vi "Parameter to Value.vi"(8 "Memory":cluster{"w":i64, "x":i64, "y":i64, "z":i64}, 11 "Parameter":string) -> (3 "Value Out":i64)   [LabVIEW 2021]
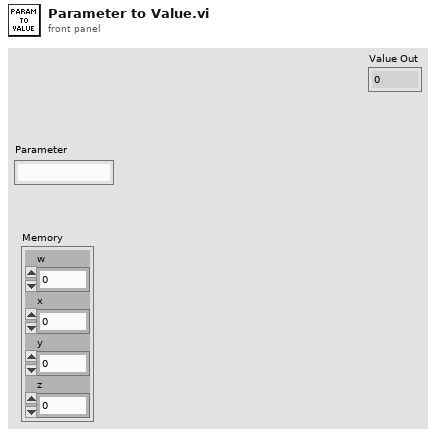
[diagram p1: front panel]
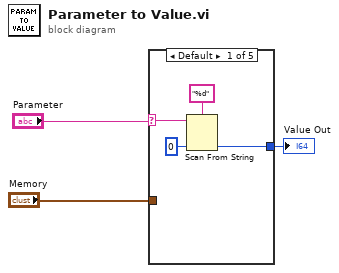
[diagram p0: block diagram]
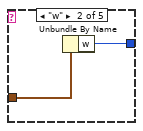
[diagram p2: hidden frame]
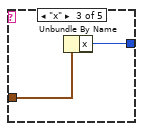
[diagram p3: hidden frame]
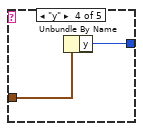
[diagram p4: hidden frame]
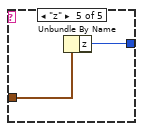
[diagram p5: hidden frame]
diagram:
  n1 = case shown="Default" "Parameter" {
    selector: "Parameter" -> [w7 _ _ _ _]
    tunnel: "Memory" -> [_ w9 w11 w13 w15]
    tunnel: [w4 w8 w10 w12 w14] -> w1
    frame Default {
      n2 = Scan From String(format string="%d", input string=w7, default 1=i64 0 ("default value 1")) -> (output 1=w4:i64)  [unwired: 2 in, 3 out]
    }
    frame "w" {
      n3 = Unbundle By Name(w9) -> ("w"=w8:i64)
    }
    frame "x" {
      n4 = Unbundle By Name(w11) -> ("x"=w10:i64)
    }
    frame "y" {
      n5 = Unbundle By Name(w13) -> ("y"=w12:i64)
    }
    frame "z" {
      n6 = Unbundle By Name(w15) -> ("z"=w14:i64)
    }
  }
  "Value Out" <- w1
